vi "MoAgSy_AgentBase_GPG_cryption.vi"(0 "HGF_Agent in":refnum<class "MoAgSy_AgentBase.lvclass">, 2 "string in":string, 5 "error in (no error)":errorcluster, 7 "reveicer array":string[](array[string]), 8 "task":enum16{"encrypt", "decrypt", "sign", "verify"}(ring), 9 "receiver":string) -> (14 "dup HGF_Agent":refnum<class "MoAgSy_AgentBase.lvclass">, 16 "String out":string, 18 "success":bool=TRUE, 19 "error out":errorcluster)   [LabVIEW 2009, in "MoAgSy_Base.lvlib" / "MoAgSy_AgentBase.lvclass"]
uses:
  MoAgSy_AgentBase.lvclass
  MoAgSy_AgentBase.lvclass/MoAgSy_AgentBase.ctl
  MoAgSy_GPG/MoAgSy_GPG.lvclass
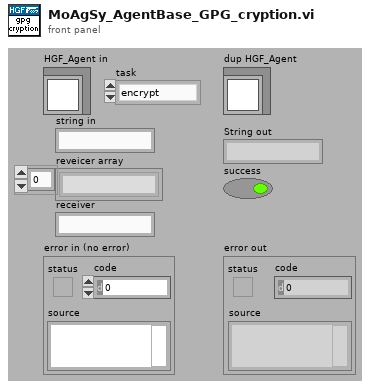
[diagram p1: front panel]
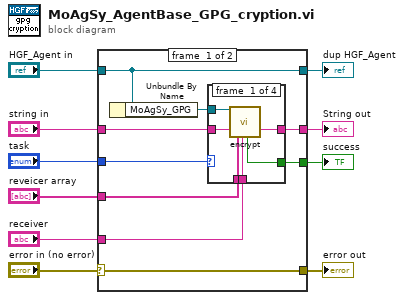
[diagram p0: block diagram]
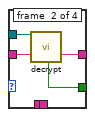
[diagram p2: hidden frame]
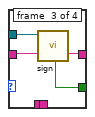
[diagram p3: hidden frame]
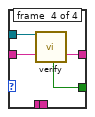
[diagram p4: hidden frame]
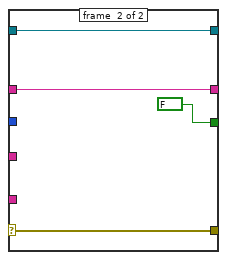
[diagram p5: hidden frame]
diagram:
  n1 = case shown="No Error" "error in (no error)" {
    selector: "error in (no error)" -> [w19 w41]
    tunnel: [w19 w41] -> w9
    tunnel: [w18 w40] -> w7
    tunnel: "HGF_Agent in" -> [w18 w40]
    tunnel: "string in" -> [w16 w39]
    tunnel: "reveicer array" -> [w15 _]
    tunnel: "receiver" -> [w14 _]
    tunnel: [w13 w39] -> w3
    tunnel: "task" -> [w12 _]
    tunnel: [w11 FALSE ("success")] -> w1
    frame #0 {
      n2 = Unbundle By Name(w18) -> ("MoAgSy_GPG"=w17:refnum<class "MoAgSy_GPG.lvclass">)
      n3 = case shown="\"encrypt\"" w12 {
        tunnel: w17 -> [w25 w29 w33 w36]
        tunnel: w16 -> [w24 w28 w32 w37]
        tunnel: w15 -> [w23 _ _ _]
        tunnel: w14 -> [w22 _ _ _]
        tunnel: [w21 w27 w31 w35] -> w13
        tunnel: [w20 w26 w30 w34] -> w11
        frame #0 {
          n4 = call-dynamic "encrypt.vi"("HGF_GPG"=w25, "string in"=w24, "reveicer array"=w23, "receiver"=w22) -> ("success"=w20:bool, "String out"=w21:string)  [unwired: 5 in, 9 out]
        }
        frame #1 {
          n5 = call-dynamic "decrypt.vi"("HGF_GPG"=w29, "string in"=w28) -> ("success"=w26:bool, "String"=w27:string)  [unwired: 6 in, 10 out]
        }
        frame #2 {
          n6 = call-dynamic "sign.vi"("HGF_GPG"=w33, "string in"=w32) -> ("success"=w30:bool, "String out"=w31:string)  [unwired: 7 in, 9 out]
        }
        frame #3 {
          n7 = call-dynamic "verify.vi"("HGF_GPG"=w36, "string in"=w37) -> ("success"=w34:bool, "String"=w35:string)  [unwired: 5 in, 11 out]
        }
      }
    }
    frame #1 {
    }
  }
  "error out" <- w9
  "dup HGF_Agent" <- w7
  "String out" <- w3
  "success" <- w1
